vi "sendMessage.vi"(8 "error in (no error)":errorcluster, 9 "data":variant, 10 "message":string, 11 "ITaskChannel in":refnum<class "ITaskChannel.lvclass">) -> (0 "error out":errorcluster, 3 "ITaskChannel out":refnum<class "ITaskChannel.lvclass">)   [LabVIEW 2023, in "TLC_Daemon.lvlib" / "ITaskChannel.lvclass"]
uses:
  ITaskChannel.lvclass
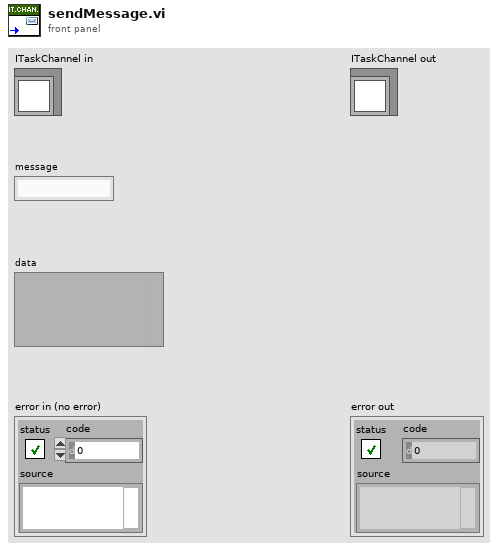
[diagram p1: front panel]
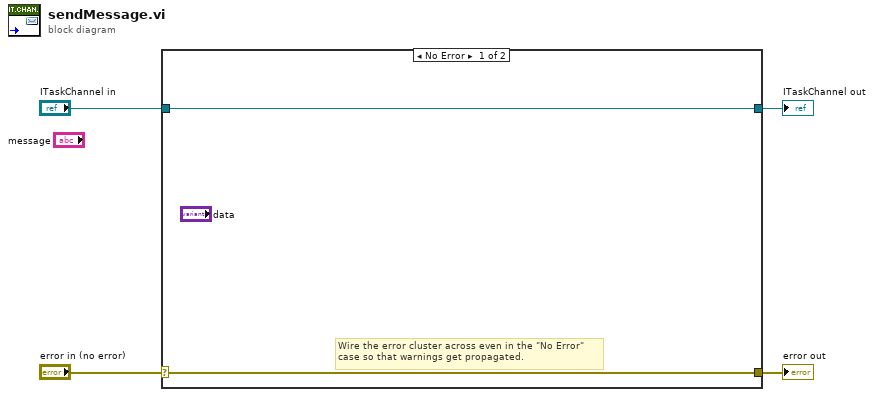
[diagram p0: block diagram]
diagram:
  n1 = case shown="No Error" "error in (no error)" {
    selector: "error in (no error)" -> [w5 w8]
    tunnel: [w5 w8] -> w3
    tunnel: [w6 w7] -> w1
    tunnel: "ITaskChannel in" -> [w6 w7]
    frame No Error {
      # "Wire the error cluster across even in the \"No Error\"\ncase so that warnings get propagated."
    }
    frame Error {
    }
  }
  "error out" <- w3
  "ITaskChannel out" <- w1
